vi "SmartSEM Remote API get Zeiss parameters.vi"(8 "error in":errorcluster, 9 "FIB":bool=TRUE, 11 "ActiveX Container":refnum<k7>(container)) -> (0 "error out":errorcluster, 1 "FIB parameters":T1 {"FIB probe current" format="%.3f"}, 2 "SEM parameters":T2, 3 "reference out":refnum<k7>)   [LabVIEW 2018]
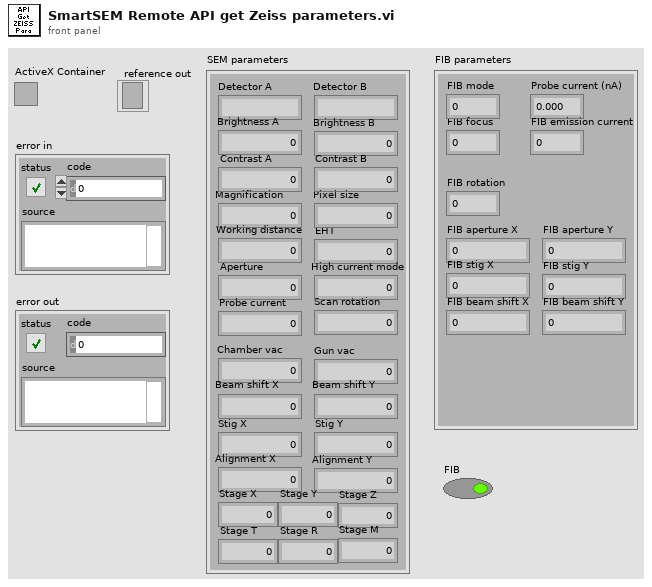
[diagram p1: front panel]
types:
  T1 = cluster{"FIB mode":u8, "FIB focus":sgl, "FIB probe current":sgl, "FIB emission current":sgl, "FIB rotation":sgl, "FIB aperture X":sgl, "FIB aperture Y":sgl, "FIB stig X":sgl, "FIB stig Y":sgl, "FIB beam shift X":sgl, "FIB beam shift Y":sgl}
  T2 = cluster{"Detector A":string, "Detector B":string, "Brightness A":sgl, "Contrast A":sgl, "Brightness B":sgl, "Contrast B":sgl, "Magnification":sgl, "Pixel size":sgl, "Working distance":sgl, "EHT":sgl, "Aperture":u8, "High current mode":u8, "Probe current":sgl, "Scan rotation":sgl, "Chamber vac":sgl, "Gun vac":sgl, "Beam shift X":sgl, "Beam shift Y":sgl, "Stig X":sgl, "Stig Y":sgl, "Alignment X":sgl, "Alignment Y":sgl, "Stage X":sgl, "Stage Y":sgl, "Stage Z":sgl, "Stage T":sgl, "Stage R":sgl, "Stage M":sgl}
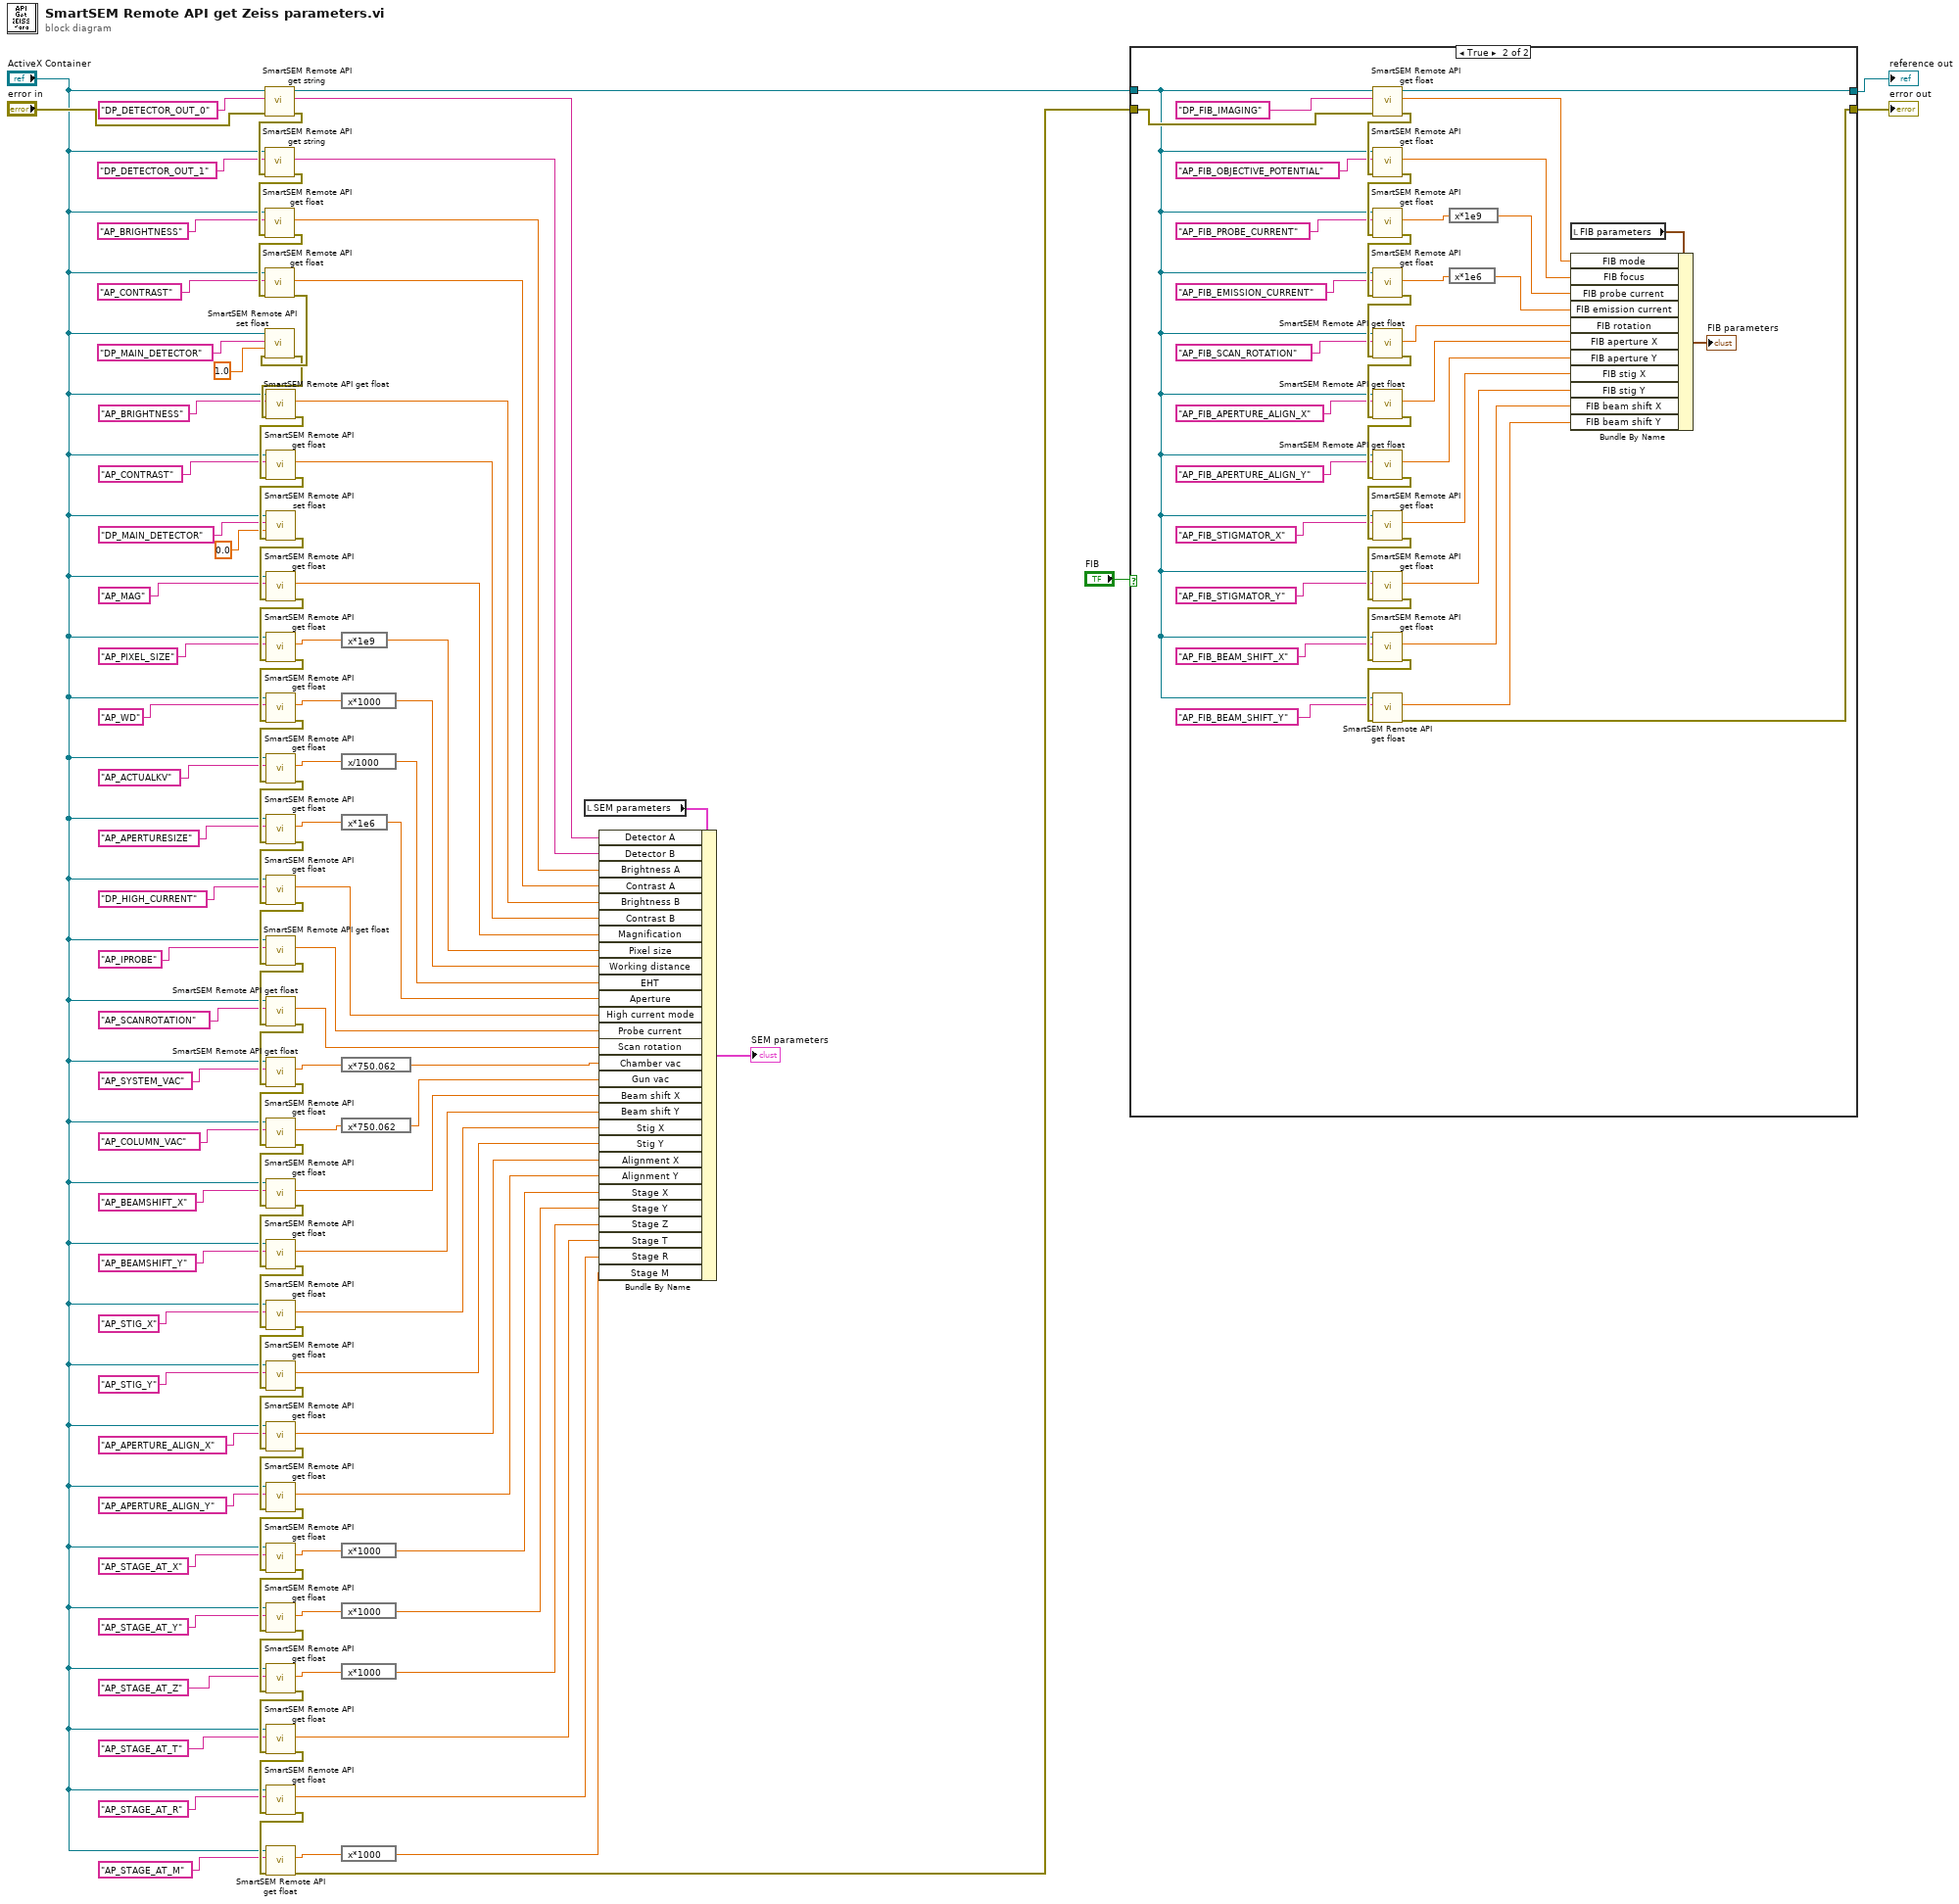
[diagram p0: block diagram]
diagram:
  n1 = call "SmartSEM Remote API get string.vi"("error in"="error in", "lpszParam"="DP_DETECTOR_OUT_0", "ActiveX Container"="ActiveX Container") -> ("error out"=w81:errorcluster, "data"=w76:string, "reference out"=w39:refnum<k7>)  [unwired: 6 in]
  n2 = call "SmartSEM Remote API get string.vi"("error in"=w81, "lpszParam"="DP_DETECTOR_OUT_1", "ActiveX Container"="ActiveX Container") -> ("error out"=w80:errorcluster, "data"=w75:string)  [unwired: 6 in, 1 out]
  n3 = call "SmartSEM Remote API get float.vi"("error in"=w80, "lpszParam"="AP_BRIGHTNESS", "ActiveX Container"="ActiveX Container") -> ("error out"=w79:errorcluster, "vValue"=w14:sgl)  [unwired: 6 in, 1 out]
  n4 = call "SmartSEM Remote API get float.vi"("error in"=w79, "lpszParam"="AP_CONTRAST", "ActiveX Container"="ActiveX Container") -> ("error out"=w69:errorcluster, "vValue"=w15:sgl)  [unwired: 6 in, 1 out]
  n5 = call "SmartSEM Remote API set float.vi"("error in"=w69, "vValue"=sgl 1.0, "lpszParam"="DP_MAIN_DETECTOR", "ActiveX Container"="ActiveX Container") -> ("error out"=w68:errorcluster)  [unwired: 6 in, 1 out]
  n6 = call "SmartSEM Remote API get float.vi"("error in"=w68, "lpszParam"="AP_BRIGHTNESS", "ActiveX Container"="ActiveX Container") -> ("error out"=w82:errorcluster, "vValue"=w16:sgl)  [unwired: 6 in, 1 out]
  n7 = call "SmartSEM Remote API get float.vi"("error in"=w82, "lpszParam"="AP_CONTRAST", "ActiveX Container"="ActiveX Container") -> ("error out"=w83:errorcluster, "vValue"=w17:sgl)  [unwired: 6 in, 1 out]
  n8 = call "SmartSEM Remote API set float.vi"("error in"=w83, "vValue"=sgl 0.0, "lpszParam"="DP_MAIN_DETECTOR", "ActiveX Container"="ActiveX Container") -> ("error out"=w84:errorcluster)  [unwired: 6 in, 1 out]
  n9 = call "SmartSEM Remote API get float.vi"("error in"=w84, "lpszParam"="AP_MAG", "ActiveX Container"="ActiveX Container") -> ("error out"=w85:errorcluster, "vValue"=w18:sgl)  [unwired: 6 in, 1 out]
  n10 = call "SmartSEM Remote API get float.vi"("error in"=w85, "lpszParam"="AP_PIXEL_SIZE", "ActiveX Container"="ActiveX Container") -> ("error out"=w86:errorcluster, "vValue"=w36:sgl)  [unwired: 6 in, 1 out]
  n11 = call "SmartSEM Remote API get float.vi"("error in"=w86, "lpszParam"="AP_WD", "ActiveX Container"="ActiveX Container") -> ("error out"=w92:errorcluster, "vValue"=w37:sgl)  [unwired: 6 in, 1 out]
  n12 = call "SmartSEM Remote API get float.vi"("error in"=w92, "lpszParam"="AP_ACTUALKV", "ActiveX Container"="ActiveX Container") -> ("error out"=w91:errorcluster, "vValue"=w38:sgl)  [unwired: 6 in, 1 out]
  n13 = call "SmartSEM Remote API get float.vi"("error in"=w91, "lpszParam"="AP_APERTURESIZE", "ActiveX Container"="ActiveX Container") -> ("error out"=w90:errorcluster, "vValue"=w33:sgl)  [unwired: 6 in, 1 out]
  n14 = call "SmartSEM Remote API get float.vi"("error in"=w90, "lpszParam"="DP_HIGH_CURRENT", "ActiveX Container"="ActiveX Container") -> ("error out"=w89:errorcluster, "vValue"=w35:sgl)  [unwired: 6 in, 1 out]
  n15 = call "SmartSEM Remote API get float.vi"("error in"=w89, "lpszParam"="AP_IPROBE", "ActiveX Container"="ActiveX Container") -> ("error out"=w88:errorcluster, "vValue"=w20:sgl)  [unwired: 6 in, 1 out]
  n16 = call "SmartSEM Remote API get float.vi"("error in"=w88, "lpszParam"="AP_SCANROTATION", "ActiveX Container"="ActiveX Container") -> ("error out"=w87:errorcluster, "vValue"=w19:sgl)  [unwired: 6 in, 1 out]
  n17 = call "SmartSEM Remote API get float.vi"("error in"=w87, "lpszParam"="AP_SYSTEM_VAC", "ActiveX Container"="ActiveX Container") -> ("error out"=w94:errorcluster, "vValue"=w34:sgl)  [unwired: 6 in, 1 out]
  n18 = call "SmartSEM Remote API get float.vi"("error in"=w94, "lpszParam"="AP_COLUMN_VAC", "ActiveX Container"="ActiveX Container") -> ("error out"=w93:errorcluster, "vValue"=w12:sgl)  [unwired: 6 in, 1 out]
  n19 = call "SmartSEM Remote API get float.vi"("error in"=w93, "lpszParam"="AP_BEAMSHIFT_X", "ActiveX Container"="ActiveX Container") -> ("error out"=w47:errorcluster, "vValue"=w11:sgl)  [unwired: 6 in, 1 out]
  n20 = call "SmartSEM Remote API get float.vi"("error in"=w47, "lpszParam"="AP_BEAMSHIFT_Y", "ActiveX Container"="ActiveX Container") -> ("error out"=w50:errorcluster, "vValue"=w10:sgl)  [unwired: 6 in, 1 out]
  n21 = call "SmartSEM Remote API get float.vi"("error in"=w50, "lpszParam"="AP_STIG_X", "ActiveX Container"="ActiveX Container") -> ("error out"=w51:errorcluster, "vValue"=w9:sgl)  [unwired: 6 in, 1 out]
  n22 = call "SmartSEM Remote API get float.vi"("error in"=w51, "lpszParam"="AP_STIG_Y", "ActiveX Container"="ActiveX Container") -> ("error out"=w52:errorcluster, "vValue"=w8:sgl)  [unwired: 6 in, 1 out]
  n23 = call "SmartSEM Remote API get float.vi"("error in"=w52, "lpszParam"="AP_APERTURE_ALIGN_X", "ActiveX Container"="ActiveX Container") -> ("error out"=w53:errorcluster, "vValue"=w7:sgl)  [unwired: 6 in, 1 out]
  n24 = call "SmartSEM Remote API get float.vi"("error in"=w53, "lpszParam"="AP_APERTURE_ALIGN_Y", "ActiveX Container"="ActiveX Container") -> ("error out"=w48:errorcluster, "vValue"=w4:sgl)  [unwired: 6 in, 1 out]
  n25 = call "SmartSEM Remote API get float.vi"("error in"=w48, "lpszParam"="AP_STAGE_AT_X", "ActiveX Container"="ActiveX Container") -> ("error out"=w49:errorcluster, "vValue"=w32:sgl)  [unwired: 6 in, 1 out]
  n26 = call "SmartSEM Remote API get float.vi"("error in"=w49, "lpszParam"="AP_STAGE_AT_Y", "ActiveX Container"="ActiveX Container") -> ("error out"=w27:errorcluster, "vValue"=w31:sgl)  [unwired: 6 in, 1 out]
  n27 = call "SmartSEM Remote API get float.vi"("error in"=w27, "lpszParam"="AP_STAGE_AT_Z", "ActiveX Container"="ActiveX Container") -> ("error out"=w28:errorcluster, "vValue"=w26:sgl)  [unwired: 6 in, 1 out]
  n28 = call "SmartSEM Remote API get float.vi"("error in"=w28, "lpszParam"="AP_STAGE_AT_T", "ActiveX Container"="ActiveX Container") -> ("error out"=w30:errorcluster, "vValue"=w5:sgl)  [unwired: 6 in, 1 out]
  n29 = call "SmartSEM Remote API get float.vi"("error in"=w30, "lpszParam"="AP_STAGE_AT_R", "ActiveX Container"="ActiveX Container") -> ("error out"=w29:errorcluster, "vValue"=w6:sgl)  [unwired: 6 in, 1 out]
  n30 = call "SmartSEM Remote API get float.vi"("error in"=w29, "lpszParam"="AP_STAGE_AT_M", "ActiveX Container"="ActiveX Container") -> ("error out"=w3:errorcluster, "vValue"=w25:sgl)  [unwired: 6 in, 1 out]
  n31 = expression code="x*1e9"(w36) -> (w105:sgl)
  n32 = expression code="x*1000"(w37) -> (w106:sgl)
  n33 = expression code="x/1000"(w38) -> (w104:sgl)
  n34 = expression code="x*1e6"(w33) -> (w96:sgl)
  n35 = expression code="x*750.062"(w34) -> (w99:sgl)
  n36 = expression code="x*750.062"(w12) -> (w98:sgl)
  n37 = expression code="x*1000"(w32) -> (w103:sgl)
  n38 = expression code="x*1000"(w31) -> (w102:sgl)
  n39 = expression code="x*1000"(w26) -> (w101:sgl)
  n40 = expression code="x*1000"(w25) -> (w100:sgl)
  n41 = local read "SEM parameters"() -> (w108:T2)
  n42 = Bundle By Name(cluster=w108, "Detector A"=w76, "Detector B"=w75, "Brightness A"=w14, "Contrast A"=w15, "Brightness B"=w16, "Contrast B"=w17, "Magnification"=w18, "Pixel size"=w105, "Working distance"=w106, "EHT"=w104, "Aperture"=w96, "High current mode"=w35, "Probe current"=w20, "Scan rotation"=w19, "Chamber vac"=w99, "Gun vac"=w98, "Beam shift X"=w11, "Beam shift Y"=w10, "Stig X"=w9, "Stig Y"=w8, "Alignment X"=w7, "Alignment Y"=w4, "Stage X"=w103, "Stage Y"=w102, "Stage Z"=w101, "Stage T"=w5, "Stage R"=w6, "Stage M"=w100) -> (→"SEM parameters":T2)
  n43 = case shown="True" "FIB" {
    tunnel: [w110 w114] -> w95
    tunnel: w39 -> [w110 w111]
    tunnel: w3 -> [w109 w113]
    tunnel: [w109 w112] -> w2
    frame False {
    }
    frame True {
      n44 = call "SmartSEM Remote API get float.vi"("error in"=w113, "lpszParam"="DP_FIB_IMAGING", "ActiveX Container"=w111) -> ("error out"=w146:errorcluster, "vValue"=w122:sgl, "reference out"=w114:refnum<k7>)  [unwired: 6 in]
      n45 = call "SmartSEM Remote API get float.vi"("error in"=w146, "lpszParam"="AP_FIB_OBJECTIVE_POTENTIAL", "ActiveX Container"=w111) -> ("error out"=w145:errorcluster, "vValue"=w123:sgl)  [unwired: 6 in, 1 out]
      n46 = call "SmartSEM Remote API get float.vi"("error in"=w145, "lpszParam"="AP_FIB_PROBE_CURRENT", "ActiveX Container"=w111) -> ("error out"=w144:errorcluster, "vValue"=w125:sgl)  [unwired: 6 in, 1 out]
      n47 = call "SmartSEM Remote API get float.vi"("error in"=w144, "lpszParam"="AP_FIB_EMISSION_CURRENT", "ActiveX Container"=w111) -> ("error out"=w143:errorcluster, "vValue"=w124:sgl)  [unwired: 6 in, 1 out]
      n48 = call "SmartSEM Remote API get float.vi"("error in"=w143, "lpszParam"="AP_FIB_SCAN_ROTATION", "ActiveX Container"=w111) -> ("error out"=w142:errorcluster, "vValue"=w121:sgl)  [unwired: 6 in, 1 out]
      n49 = call "SmartSEM Remote API get float.vi"("error in"=w142, "lpszParam"="AP_FIB_APERTURE_ALIGN_X", "ActiveX Container"=w111) -> ("error out"=w137:errorcluster, "vValue"=w120:sgl)  [unwired: 6 in, 1 out]
      n50 = call "SmartSEM Remote API get float.vi"("error in"=w137, "lpszParam"="AP_FIB_APERTURE_ALIGN_Y", "ActiveX Container"=w111) -> ("error out"=w138:errorcluster, "vValue"=w119:sgl)  [unwired: 6 in, 1 out]
      n51 = call "SmartSEM Remote API get float.vi"("error in"=w138, "lpszParam"="AP_FIB_STIGMATOR_X", "ActiveX Container"=w111) -> ("error out"=w139:errorcluster, "vValue"=w118:sgl)  [unwired: 6 in, 1 out]
      n52 = call "SmartSEM Remote API get float.vi"("error in"=w139, "lpszParam"="AP_FIB_STIGMATOR_Y", "ActiveX Container"=w111) -> ("error out"=w140:errorcluster, "vValue"=w117:sgl)  [unwired: 6 in, 1 out]
      n53 = call "SmartSEM Remote API get float.vi"("error in"=w140, "lpszParam"="AP_FIB_BEAM_SHIFT_X", "ActiveX Container"=w111) -> ("error out"=w141:errorcluster, "vValue"=w116:sgl)  [unwired: 6 in, 1 out]
      n54 = call "SmartSEM Remote API get float.vi"("error in"=w141, "lpszParam"="AP_FIB_BEAM_SHIFT_Y", "ActiveX Container"=w111) -> ("error out"=w112:errorcluster, "vValue"=w115:sgl)  [unwired: 6 in, 1 out]
      n55 = expression code="x*1e9"(w125) -> (w148:sgl)
      n56 = expression code="x*1e6"(w124) -> (w147:sgl)
      n57 = local read "FIB parameters"() -> (w150:T1)
      n58 = Bundle By Name(cluster=w150, "FIB mode"=w122, "FIB focus"=w123, "FIB probe current"=w148, "FIB emission current"=w147, "FIB rotation"=w121, "FIB aperture X"=w120, "FIB aperture Y"=w119, "FIB stig X"=w118, "FIB stig Y"=w117, "FIB beam shift X"=w116, "FIB beam shift Y"=w115) -> (→"FIB parameters":T1)
    }
  }
  "error out" <- w2
  "reference out" <- w95
